vi "Launcher.vi"() -> ()   [LabVIEW 2021, in "Echo Broadcast Test With Server Manager.lvlib"]
uses:
  Echo Broadcast Test With Server Manager.lvlib
  WS Test Server Subscriber/WS Test Server Subscriber.lvclass
  C:/Program Files/National Instruments/LabVIEW 2021/vi.lib/ActorFramework/Actor/Actor.lvclass
  WebSocket Actor/WebSocket Server Manager/WebSocket Server Manager.lvclass
  WS Test Server Subscriber/WS Test Server Subscriber.lvclass/WS Test Server Subscriber.ctl
  WS Test Client Subscriber/WS Test Client Subscriber.lvclass
  <vilib>/ActorFramework/Message Enqueuer/Message Enqueuer.lvclass/Message Enqueuer.ctl
  WS Test Server Subscriber/properties/Write WebSocket Server Manager Enqueuer.vi
  <vilib>/ActorFramework/Message Enqueuer/Enqueue.vi
  <vilib>/ActorFramework/Stop Msg/Stop Msg.lvclass
  C:/Program Files/National Instruments/LabVIEW 2021/vi.lib/ActorFramework/Message/Message.lvclass
  <vilib>/Utility/LVClass/Get LV Class Name.vi
  <resource>/AFDebug/Generate Trace for Message.vi
  <vilib>/ActorFramework/Message Priority Queue/Priority Enqueue.vi
  <vilib>/ActorFramework/Actor/Actor.lvclass
panel:
  in  "Stop Actors":bool
  in  "Number of Clients":i32=3
  out "error out":errorcluster
  # "In this example we will use the Server Manager Actor Infrastructure to launch a WebSocket server and we will illustrate a bidirectional communication between the WebSocket server and clients. \nWe launch one server that will define the /echo/ service. Then a user selectable number of clients can be launched. From such clients messages to the servers can be sent on the specified service. The server will echo back the message to the clients. The server can broadcast messages to the clients. One can choose to send a series of messages at a certain time frequency. \nInstructions to execute the example;\n1. Run this VI\n2. Wait that the Server and Client GUI appear\n3. use the GUIs to exchange messages\n4. Stop the actors from this VI"
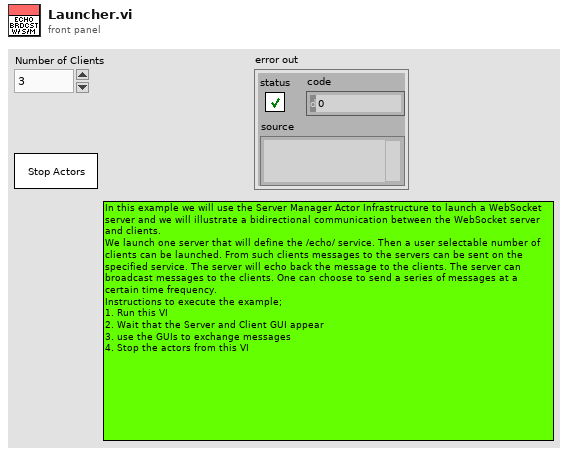
[diagram p1: front panel]
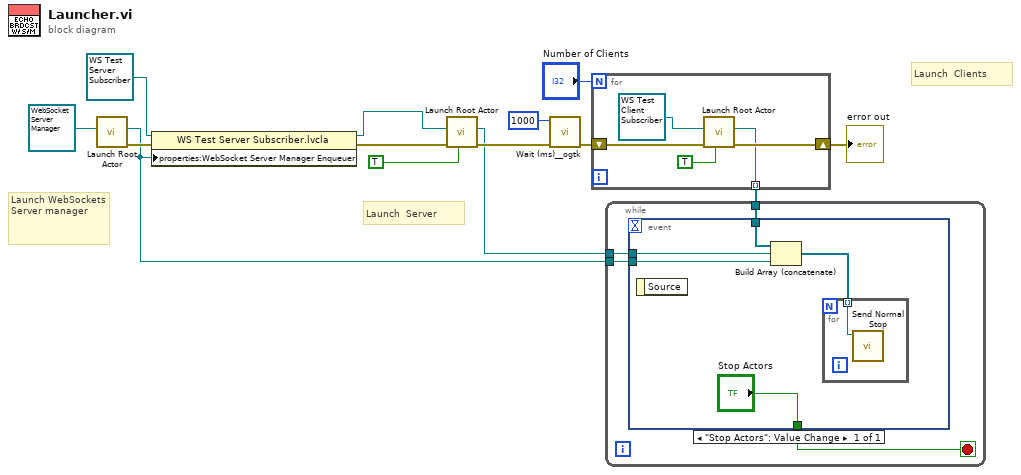
[diagram p0: block diagram]
diagram:
  # "Launch  Clients"
  # "Launch  Server"
  # "Launch WebSockets Server manager"
  n1 = call <vilib>:"Launch Root Actor.vi"("Actor"=refnum<class "WebSocket Server Manager.lvclass"> refnum ("WebSocket Actors.lvlib:WebSocket Server Manager.lvclass")) -> ("error out"=w8:errorcluster, "Actor's Enqueuer"=w4:refnum<class "Message Enqueuer.lvclass">)  [unwired: 9 in]
  n2 = property class="WS Test Server Subscriber.lvcla"(reference=refnum<class "WS Test Server Subscriber.lvclass"> refnum ("WS Full LabVIEW Test.lvlib:WS Test Server.lvclass"), error in=w8, "properties:WebSocket Server Manager Enqueuer"=w4) -> (reference out=w9:refnum<class "WS Test Server Subscriber.lvclass">, error out=w2:errorcluster)
  n3 = call <vilib>:"Launch Root Actor.vi"("Open Actor Core front panel? (F)"=TRUE, "error in (no error)"=w2, "Actor"=w9) -> ("error out"=w12:errorcluster, "Actor's Enqueuer"=w3:refnum<class "Message Enqueuer.lvclass">)  [unwired: 7 in]
  n4 = call <userlib>:"Wait (ms)__ogtk.vi"("error in (no error)"=w12, "milliseconds to wait"=u32 1000) -> ("error out"=w7:errorcluster)  [unwired: 8 in, 1 out]
  n5 = for {
    N: "Number of Clients" -> [_]
    shift-right: [w16] -> w11
    shift-left: w7 -> [w17]
    tunnel: [w15] -> w1 mode=indexing
    n6 = call <vilib>:"Launch Root Actor.vi"("Open Actor Core front panel? (F)"=TRUE, "error in (no error)"=w17, "Actor"=refnum<class "WS Test Client Subscriber.lvclass"> refnum ("WS Full LabVIEW Test.lvlib:WS Test Client.lvclass")) -> ("error out"=w16:errorcluster, "Actor's Enqueuer"=w15:refnum<class "Message Enqueuer.lvclass">)  [unwired: 7 in]
  }
  "error out" <- w11
  n7 = while {
    tunnel: w4 -> [w23]
    tunnel: w3 -> [w21]
    tunnel: w1 -> [w20]
    stop <- w22 stop-if-true
    n8 = event shown="[0] \"Stop Actors\": Value Change" {
      selector: _ -> [_]
      dyn-events: _ -> [_]
      timeout: _ -> [_]
      tunnel: w23 -> [w28]
      tunnel: ["Stop Actors"] -> w22
      tunnel: w21 -> [w25]
      tunnel: w20 -> [w24]
      event "Stop Actors": Value Change {
        n9 = event-data() -> ()  [unwired: 1 in, 1 out]
        n10 = Build Array (concatenate)(w24, w25, w28) -> (w26:refnum<class "Message Enqueuer.lvclass">[])
        n11 = for {
          tunnel: w26 -> [w29] mode=indexing
          n12 = call <vilib>:"Send Normal Stop.vi"("Message Enqueuer"=w29) -> ()  [unwired: 10 in, 1 out]
        }
      }
    }
  }
